vi "PADMINI_BOOLIAN_ARRAY.vi"(10 "Array in 2":string[](array[string]), 11 "Array in":string[](array[string])) -> (3 "Array out":string[](array[string]))   [LabVIEW 2017]
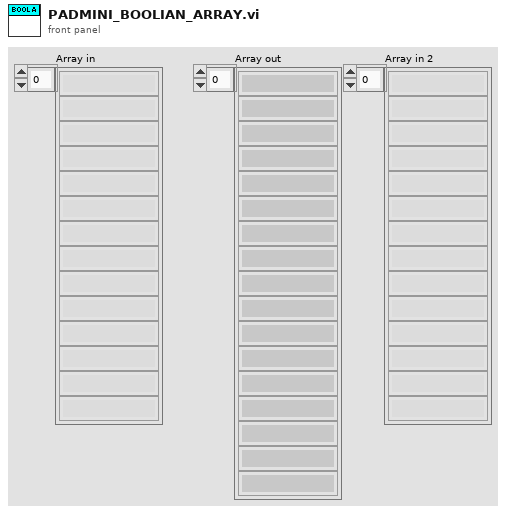
[diagram p1: front panel]
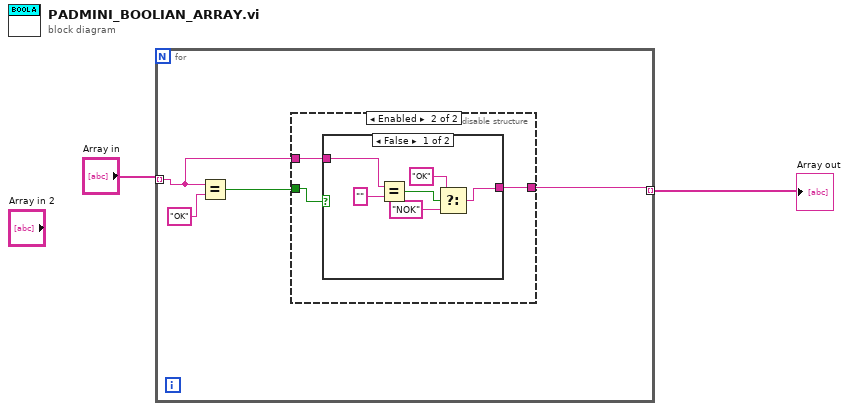
[diagram p0: block diagram]
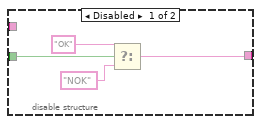
[diagram p2: hidden frame]
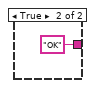
[diagram p3: hidden frame]
diagram:
  n1 = for {
    tunnel: "Array in" -> [w3] mode=indexing
    tunnel: [w6] -> w2 mode=indexing
    n2 = Equal?(x=w3, y="OK") -> (x = y?=w4:bool)
    n3 = disable-structure shown="Enabled" {
      disable-tunnel: [w8 w12] -> w6
      disable-tunnel: w4 -> [w7 w13]
      disable-tunnel: w3 -> [_ w11]
      frame Disabled {
        n4 = Select(t="OK", s=w7, f="NOK") -> (s? t:f=w8:string)
      }
      frame Enabled {
        n5 = case shown="False" w13 {
          tunnel: [w14 "OK" ("f")] -> w12
          tunnel: w11 -> [w19 _]
          frame False {
            n6 = Equal?(x=w19, y="") -> (x = y?=w17:bool)
            n7 = Select(t="OK", s=w17, f="NOK") -> (s? t:f=w14:string)
          }
          frame True {
          }
        }
      }
    }
  }
  "Array out" <- w2
